vi "Edycja Wykres 1.vi"(8 "error in (no error)":errorcluster, 10 "Data in":T3) -> (0 "error out":errorcluster)   [LabVIEW 2014]
doc: "Program do edycji wykresów\ndodaje kursory, liczy odległość między kursorami pomiarowymi"
uses:
  Kontrolki/GUI/Wysw_kursorow_silver.ctl
  Kontrolki/Przetwarzanie/Kanaly.ctl
  Kontrolki/GUI/fx_przycisk.ctl
  Kontrolki/GUI/Edycja_blokowanie_free.ctl
  Kontrolki/Debug/Debug SigParam.ctl
  Kontrolki/Debug/DebugTyp.ctl
  <vilib>/Utility/miscctls.llb/LVCursorListTypeDef.ctl
  <vilib>/Utility/miscctls.llb/LVPointTypeDef.ctl
  Kontrolki/GUI/Edycja Leg Ctrl.ctl
  Kontrolki/FVGs/FVG akcje podstawowa.ctl
  <vilib>/measure/NI_MABase.lvlib
panel:
  out "Cluster":T1
  in  "Zablokowane free out":T2[](array[typedef])
  in  "Array":T4(array[cluster])=[{"signal type"=enum."Sine Wave", "frequency"=10.0, "amplitude"=2.0}, {"signal type"=enum."Sine Wave", "frequency"=13.0, "amplitude"=1.0}, {"signal type"=enum."Sine Wave", "frequency"=7.0, "amplitude"=1.0}, {"signal type"=enum."Sine Wave", "frequency"=5.0, "amplitude"=3.0}] {"amplitude" format="%0.2p"; "frequency" format="%0.2p"}
  in  "Kursory":i32(listbox)
  in  "Tab Control":T5(tab)
  out "Wykres 1":waveform(dbl)[](graph)
  out "Wykres 3":waveform(dbl)[](graph)
  out "Wykres 2":waveform(dbl)[](graph)
  out "XY Graph":cluster{"Y":dbl[], "Y":dbl[]}(graph)
  in  "Przebieg Y":string(combo)
  in  "Przebieg X":string(combo)
  out "Parametry out":T6
  out "Data in 2":T3
  out "Przebiegi Wfm":waveform(dbl)[](array[waveform])
  in  "KursOkno":bool
  in  "Edytuj_kur":bool
  in  "Funkcja":T8
  in  "Zapisz rys":bool
  in  "Save Wykres":bool
  in  "Pomiarowe Kursor":bool
  in  "Remove Kursor":bool
  in  "Add Kursor":bool
  in  "Stop":bool
  # "UWAGA!"
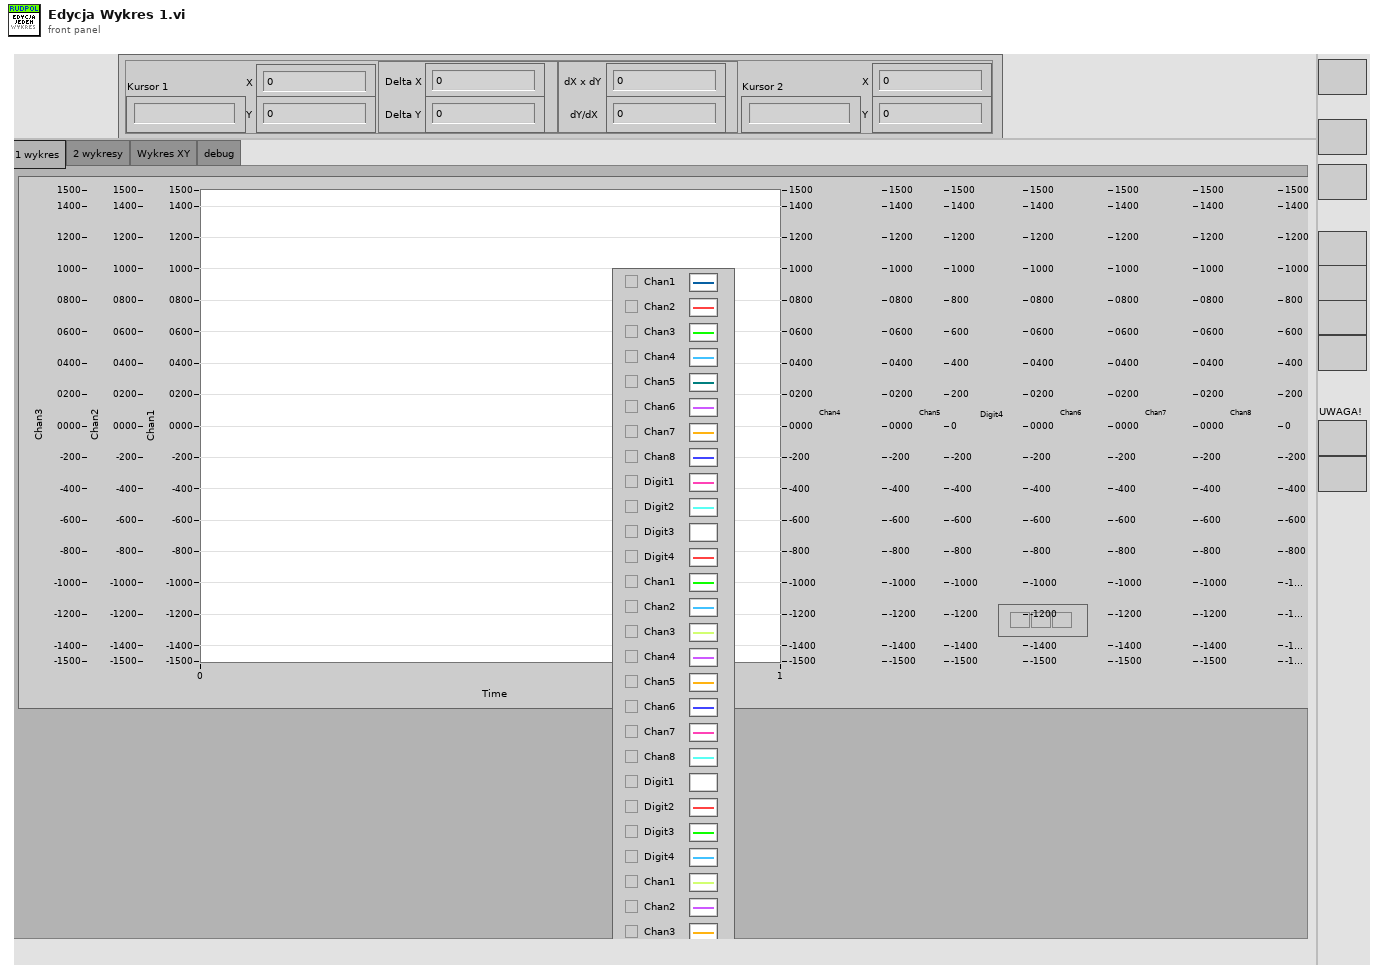
[diagram p1: front panel]
types:
  T1 = typedef "Wysw_kursorow_silver.ctl" = cluster{"Nazwa.1":string, "Nazwa.2":string, "Pos.X1":dbl, "Pos.Y1":dbl, "Delta.X":dbl, "Delta.Y":dbl, "Pos.X2":dbl, "Pos.Y2":dbl, "iloczyn dXY":dbl, "IlorazdYX":dbl}
  T2 = typedef "Edycja_blokowanie_free.ctl" = cluster{"Pozycja Y":dbl, "Pozycja X":dbl, "BlokujX":bool, "BlokujY":bool, "Zablokowane":i32}
  T3 = typedef "Kanaly.ctl" = cluster{"Analogowe":waveform(dbl)[], "Cyfrowe":waveform(dbl)[], "Zwarcie":waveform(dbl)[], "Enkoder":waveform(dbl)[]}
  T4 = cluster{"signal type":enum16{"Sine Wave", "Triangle Wave", "Square Wave", "Sawtooth Wave"}, "frequency":dbl, "amplitude":dbl}[]
  T5 = enum32{"1 wykres", "2 wykresy", "Wykres XY", "debug"}
  T6 = typedef "Debug SigParam.ctl" = cluster{"Analog":T7, "Digital":T7, "Enkoder":T7}
  T7 = typedef "DebugTyp.ctl" = cluster{"Liczba Kan":i32, "Nazwy":string[], "Rozm":i32, "dt":dbl}
  T8 = typedef "fx_przycisk.ctl" = bool
  T9 = enum16{"Sine Wave", "Triangle Wave", "Square Wave", "Sawtooth Wave"}
  T10 = typedef "Edycja Leg Ctrl.ctl" = cluster{"Leg 1":bool, "Leg 2":bool, "Leg 3":bool}
  T11 = typedef "LVPointTypeDef.ctl" = cluster{"Horizontal":i16, "Vertical":i16}
  T12 = typedef "FVG akcje podstawowa.ctl" = enum16{"GET", "SET"}
  T13 = typedef "LVCursorListTypeDef.ctl" = cluster{"Name":string, "Color":u32, "Style":u8, "Point Style":u8, "Name Visible":bool, "Allow Drag":bool, "Cursor Mode":u32, "Plot":i32, "Index":i32, "Position":cluster{"X":dbl, "Y":dbl}, "X Scale":u32, "Y Scale":u32, "Watch Plots":i32[], "Watch All Plots":bool, "Plot Area":i32, "Label Offset":cluster{"X":dbl, "Y":dbl}}[]
  T14 = typedef "LVBoundsTypeDef.ctl" = cluster{"Width":u32, "Height":u32}
  T15 = typedef "dwa_przebiegi_.ctl" = cluster{"Plot1":i32, "Plot2":i32}
  T16 = typedef "LVPoint32TypeDef.ctl" = cluster{"Horizontal":i32, "Vertical":i32}
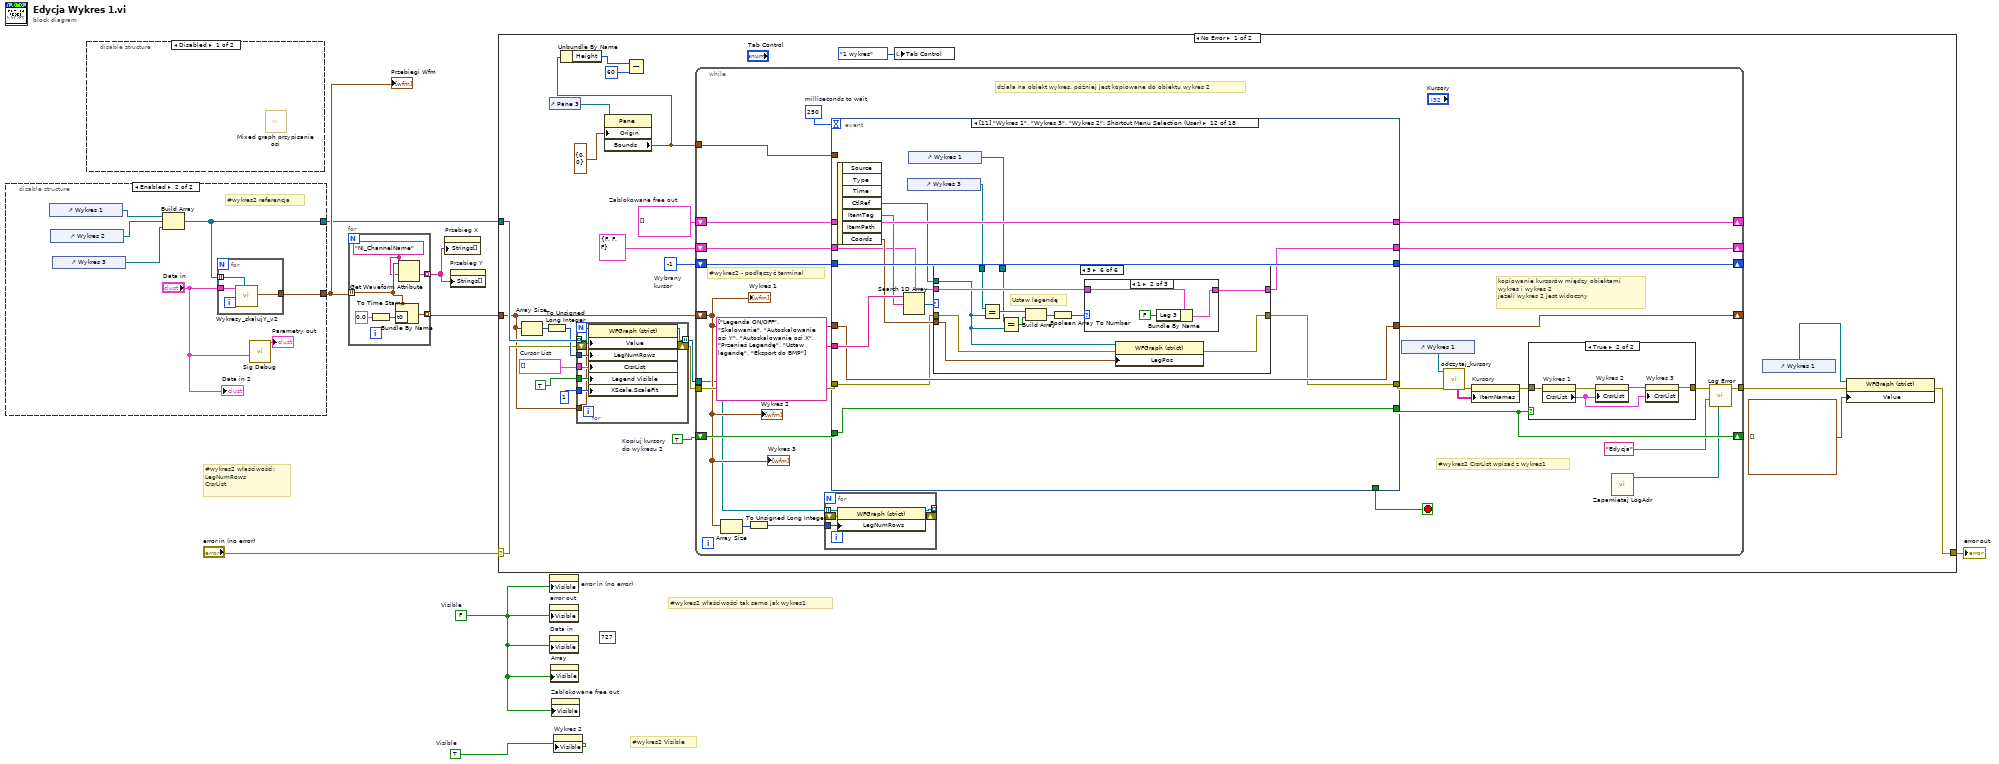
[diagram p0: block diagram]
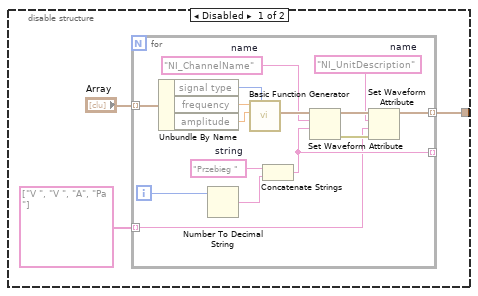
[diagram p3: hidden frame]
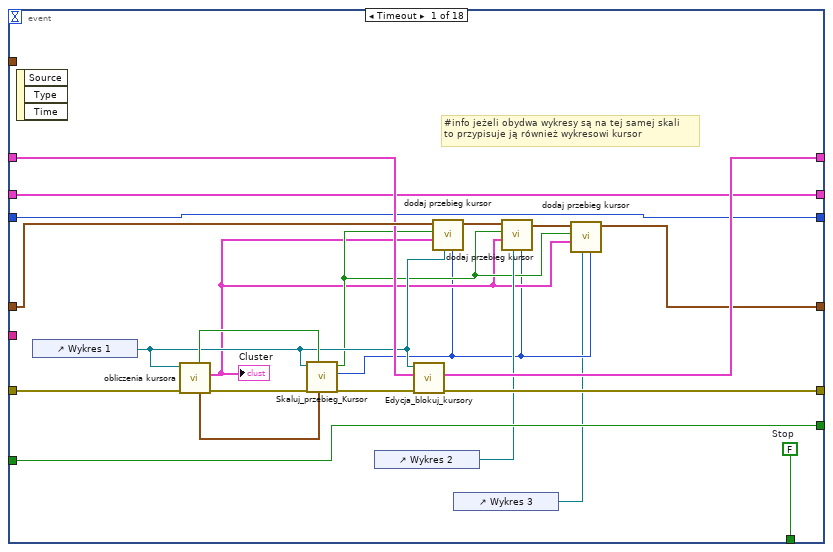
[diagram p5: hidden frame]
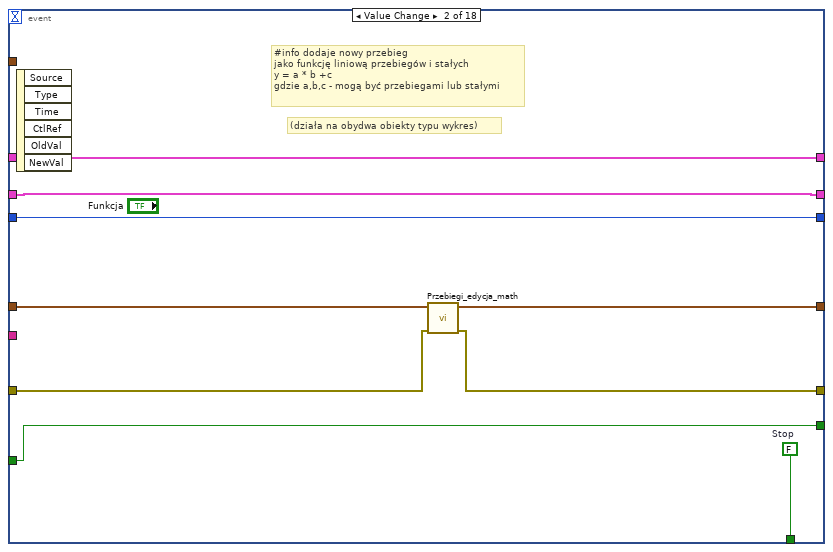
[diagram p6: hidden frame]
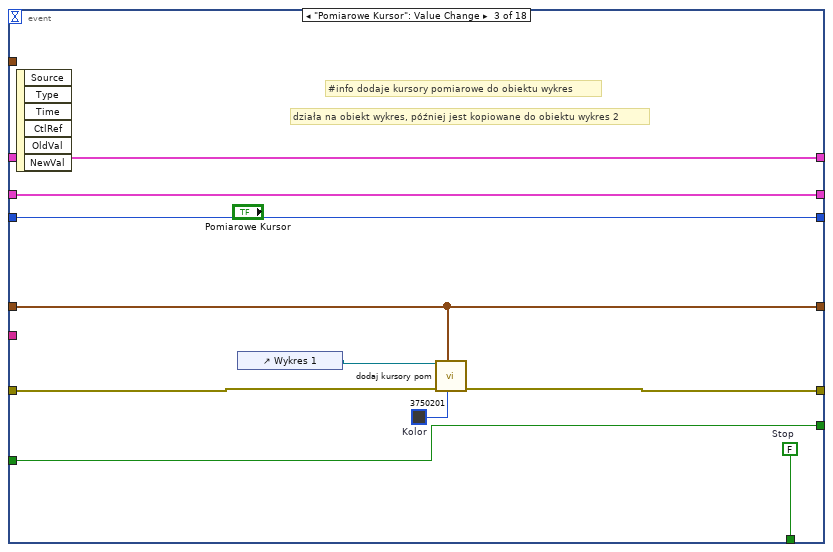
[diagram p7: hidden frame]
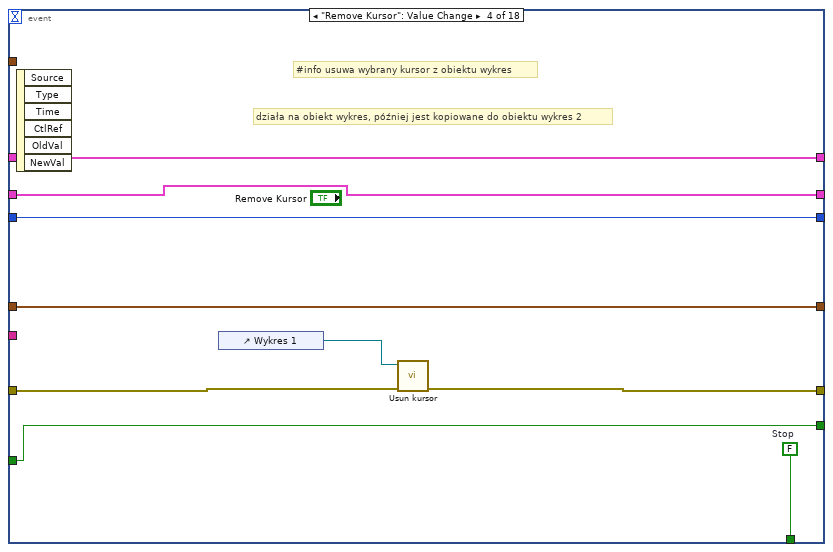
[diagram p8: hidden frame]
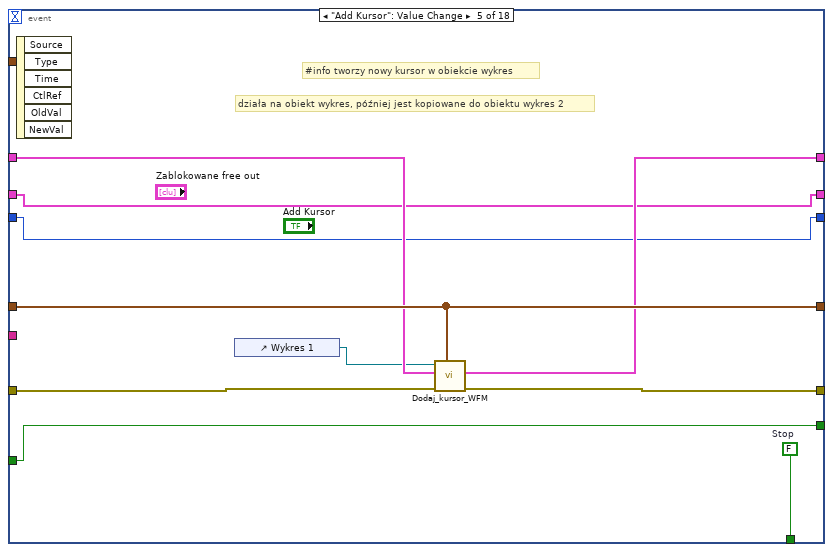
[diagram p9: hidden frame]
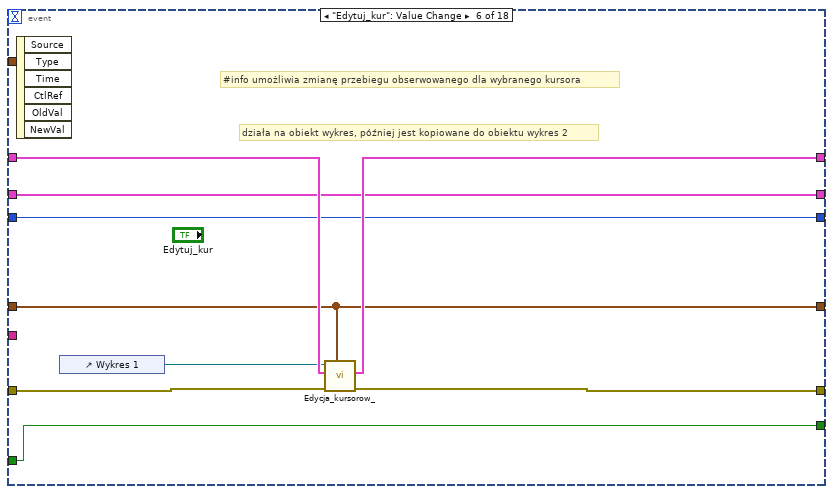
[diagram p10: hidden frame]
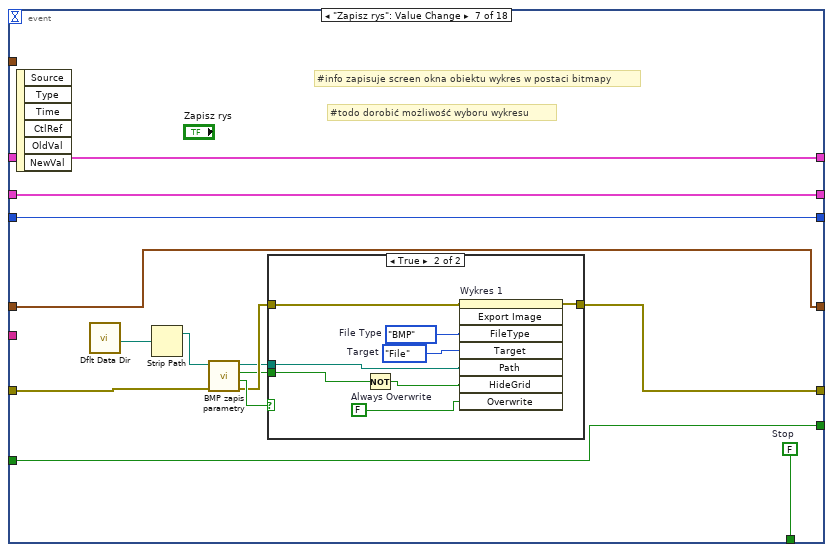
[diagram p11: hidden frame]
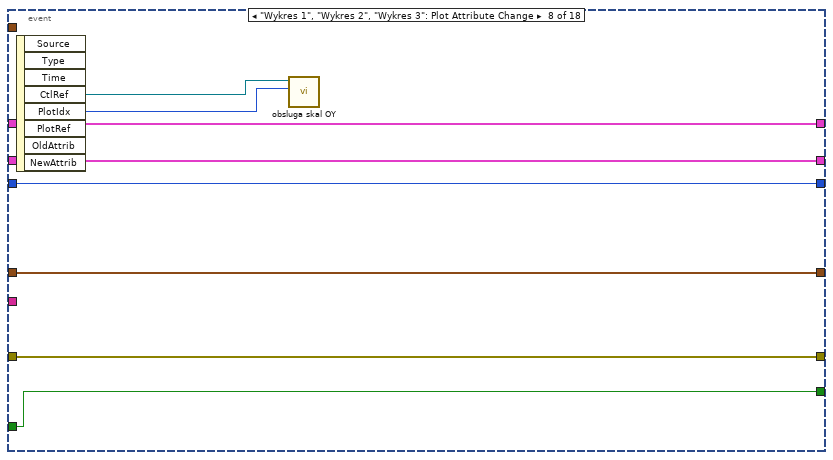
[diagram p13: hidden frame]
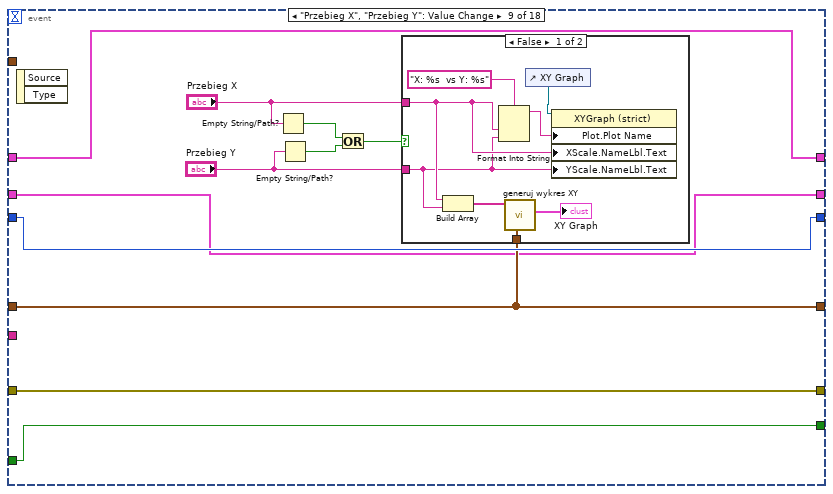
[diagram p14: hidden frame]
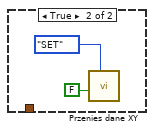
[diagram p15: hidden frame]
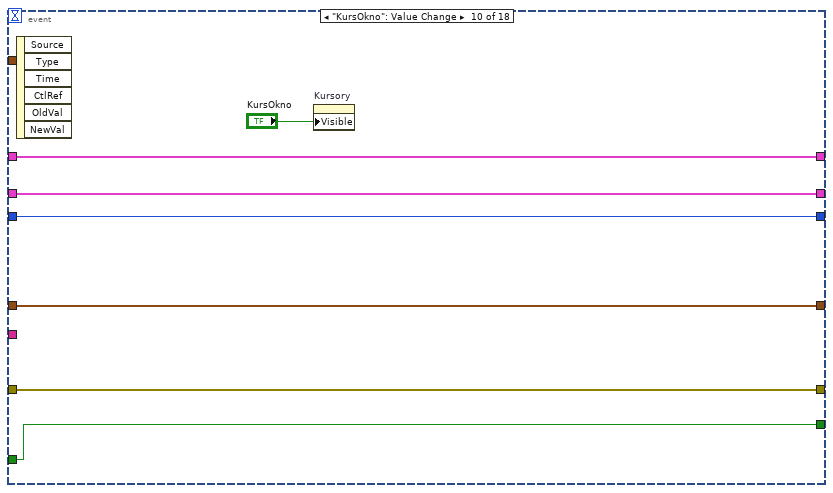
[diagram p16: hidden frame]
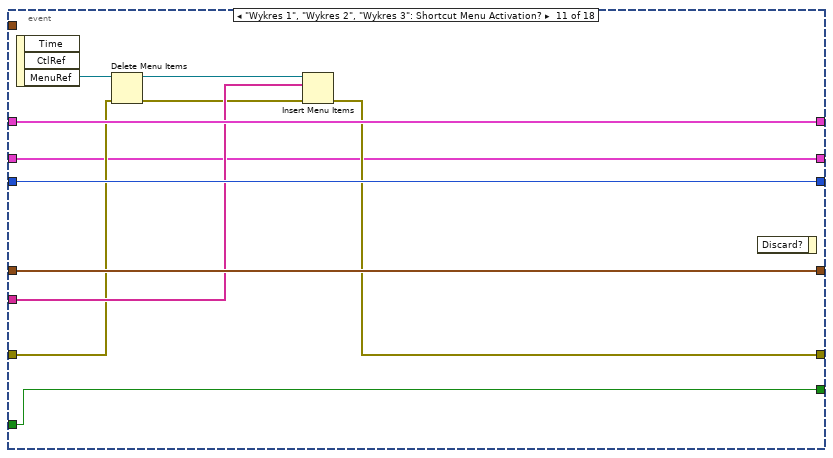
[diagram p17: hidden frame]
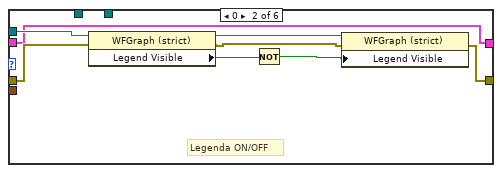
[diagram p19: hidden frame]
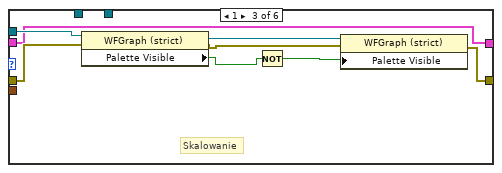
[diagram p20: hidden frame]
diagram:
  w3 = TRUE  # Visible
  (unwired) u32 727 ("Plot Area:Size:Width")
  w4 = FALSE  # Visible
  # "#wykres2 właściwości:\nLegNumRows\nCrsrList"
  # "#wykres2 Visible"
  # "#wykres2 właściwości tak samo jak wykres1"
  n1 = disable-structure shown="Enabled" {
    disable-tunnel: [w10 w28] -> w6
    disable-tunnel: [_ w27] -> w1
    frame Disabled {
      n2 = for {
        tunnel: "Array" -> [w23] mode=indexing
        tunnel: [w14] -> w10 mode=indexing
        tunnel: [w17] -> _ mode=indexing
        tunnel: string[] ["V ", "V ", "A", "Pa "] -> [w12] mode=indexing
        i -> [w18]
        w13 = "NI_UnitDescription"  # name
        w20 = "Przebieg "  # string
        w21 = "NI_ChannelName"  # name
        n3 = Unbundle By Name(w23) -> ("signal type"=w26:T9, "frequency"=w25:dbl, "amplitude"=w24:dbl)
        n4 = Number To Decimal String(number=w18) -> (decimal integer string=w19:string)  [unwired: 1 in]
        n5 = call <vilib>:"Basic Function Generator.vi"("signal type"=w26, "amplitude"=w24, "frequency"=w25) -> ("signal out"=w22:waveform(dbl))  [unwired: 6 in, 2 out]
        n6 = Concatenate Strings(w20, w19) -> (w17:string)
        n7 = Set Waveform Attribute(5:w17, 6:w21, 7:w22) -> (0:w16:errorcluster, 3:w15:waveform(dbl))  [unwired: 1 in, 1 out]
        n8 = Set Waveform Attribute(4:w16, 5:w12, 6:w13, 7:w15) -> (3:w14:waveform(dbl))  [unwired: 2 out]
      }
    }
    frame Enabled {
      # "#wykres2 referencja"
      n9 = control-ref of="Wykres 1"() -> (w31:refnum<vi>)
      n10 = control-ref of="Wykres 2"() -> (w30:refnum<vi>)
      n11 = control-ref of="Wykres 3"() -> (w29:refnum<vi>)
      n12 = Build Array(w31, w30, w29) -> (w27:refnum<vi>[])
      n13 = for {
        tunnel: "Data in" -> [w36]
        tunnel: [w35] -> w28
        tunnel: w27 -> [w34] mode=indexing
        n14 = call "Wykresy_skalujY_v2.vi"("Wvm Ref in"=w34, "Data in"=w36) -> ("Przebiegi Wfm"=w35:waveform(dbl)[])  [unwired: 7 in, 2 out]
      }
      n15 = call "Sig Debug.vi"("Kanaly in"="Data in") -> ("Parametry out"=→"Parametry out":T6)  [unwired: 8 in, 2 out]
      "Data in 2" <- "Data in"
    }
  }
  "Przebiegi Wfm" <- w6
  n16 = disable-structure shown="Disabled" {
    frame Disabled {
      n17 = call "Mixed graph przypisanie osi.vi"() -> ()  [unwired: 9 in, 3 out]
    }
    frame Enabled {
    }
  }
  n18 = for {
    tunnel: w6 -> [w39] mode=indexing
    tunnel: [w42] -> w5 mode=indexing
    tunnel: [w37] -> w2 mode=indexing
    w38 = "NI_ChannelName" ("name")
    n19 = To Time Stamp(1:0.0) -> (0:w40:timestamp)
    n20 = Bundle By Name(cluster=w39, "t0"=w40) -> (w42:waveform(dbl))
    n21 = Get Waveform Attribute(5:w38, 6:w38, 7:w39) -> (1:w37:string)  [unwired: 1 in, 3 out]
  }
  n22 = property on="Przebieg X" class="CmbBox"("Strings[]"=w2) -> ()  [unwired: 2 in, 2 out]
  n23 = property on="Przebieg Y" class="CmbBox"("Strings[]"=w2) -> ()  [unwired: 2 in, 2 out]
  n24 = case shown="No Error" "error in (no error)" {
    selector: "error in (no error)" -> [w50 w420]
    tunnel: [w61 w420] -> w7
    tunnel: w5 -> [w44 _]
    tunnel: w1 -> [w52 _]
    frame No Error {
      w63 = TRUE  # Kopiuj kursory do wykresu 2
      w64 = -1  # Wybrany kursor
      w65 = T2[] []  # Zablokowane free out
      w48 = T13 []  # Cursor List
      n25 = Array Size(array=w44) -> (size(s)=w66:i32)
      n26 = To Unsigned Long Integer(number=w66) -> (unsigned 32bit integer=w51:u32)
      n27 = control-ref of="Pane 3"() -> (w59:refnum<vi>)
      n28 = for {
        tunnel: w52 -> [w74] mode=indexing
        tunnel: w51 -> [w73]
        shift-right: [w72] -> w49
        shift-left: w50 -> [_]
        tunnel: w48 -> [w71]
        tunnel: [w70] -> w47 mode=indexing
        tunnel: u8 1 ("X Scale.Scale Fit") -> [w69]
        tunnel: TRUE ("Legend:Visible") -> [w68]
        tunnel: w44 -> [w67]
        n29 = property class="WFGraph (strict)"(reference=w74, "Value"=w67, "LegNumRows"=w73, "CrsrList"=w71, "Legend Visible"=w68, "XScale.ScaleFit"=w69) -> (reference out=w70:refnum<vi>, error out=w72:errorcluster)  [unwired: 1 in]
      }
      n30 = property class="Pane"(reference=w59, "Origin"=T11 {"Horizontal"=0, "Vertical"=0}) -> ("Bounds"=w56:T14)  [unwired: 1 in, 2 out]
      n31 = Unbundle By Name(w56) -> ("Height"=w55:u32)
      n32 = Subtract(x=w55, y=u32 60) -> ()  [unwired: 1 out]
      n33 = while {
        tunnel: w49 -> [w101]
        tunnel: [w85] -> w62
        shift-right: [w98] -> _
        shift-left: w44 -> [w79]
        shift-right: [w97] -> _
        shift-left: w65 -> [w96]
        shift-right: [w91] -> _
        shift-left: w64 -> [w92]
        shift-right: [w88] -> _
        shift-left: w63 -> [w89]
        tunnel: w56 -> [w83]
        tunnel: w47 -> [w77]
        shift-right: [w75] -> _
        shift-left: T10 {"Leg 1"=FALSE, "Leg 2"=FALSE, "Leg 3"=FALSE} ("Legenda") -> [w76]
        stop <- w99 stop-if-true
        w100 = 250  # milliseconds to wait
        # "#wykres2 CrsrList wpisać z wykres1"
        # "#wykres2 - podłączyć terminal"
        # "kopiowanie kursorów między obiektami\nwykres i wykres 2\njeżeli wykres 2 jest widoczny"
        # "działa na obiekt wykres, później jest kopiowane do obiektu wykres 2"
        n34 = Array Size(array=w79) -> (size(s)=w87:i32)
        n35 = To Unsigned Long Integer(number=w87) -> (unsigned 32bit integer=w78:u32)
        n36 = for {
          tunnel: w77 -> [w106] mode=indexing
          tunnel: w78 -> [w105]
          shift-right: [w103] -> _
          shift-left: _ -> [w104]
          tunnel: [w102] -> _ mode=indexing
          n37 = property class="WFGraph (strict)"(reference=w106, error in=w104, "LegNumRows"=w105) -> (reference out=w102:refnum<vi>, error out=w103:errorcluster)
        }
        n38 = event shown="[11] \"Wykres 1\", \"Wykres 3\", \"Wykres 2\": Shortcut Menu Selection (User)" {
          selector: _ -> [_ _ _ _ _ _ _ _ _ _ _ _ _ _ _ _ _ _]
          dyn-events: _ -> [_ _ _ _ _ _ _ _ _ _ _ _ _ _ _ _ _ _]
          timeout: w100 -> [_ _ _ _ _ _ _ _ _ _ _ _ _ _ _ _ _ _]
          tunnel: w79 -> [w131 w142 w150 w158 w170 w176 w185 w210 w213 w238 w250 w258 w340 w359 w368 w378 w411 w417]
          tunnel: w101 -> [w133 w140 w152 w161 w171 w178 w191 w211 w222 w239 w242 w256 w345 w360 w363 _ w412 w418]
          tunnel: [w126 w139 w151 w160 w166 w177 w194 w211 w222 w239 w241 w255 w344 w360 w362 w375 w412 w418] -> w94
          tunnel: [w132 w138 w148 w159 w169 _ w193 _ _ _ _ _ _ _ w367 _ _ "Stop"] -> w99
          tunnel: [w119 w141 w150 w158 w170 w176 w185 w210 w213 w238 w250 w258 w340 w359 w368 w378 w411 w417] -> w98
          tunnel: [w128 w137 w147 w157 w167 w179 w184 w209 w221 w237 w249 w265 w349 w358 w366 w377 w410 w416] -> w97
          tunnel: w96 -> [w129 w137 w147 w157 w168 w180 w184 w209 w221 w237 w249 w265 w349 w358 w366 w377 w410 w416]
          tunnel: w92 -> [w124 w136 w146 w156 w165 w175 w183 w208 w220 w236 w248 w264 w348 _ w365 w374 _ w415]
          tunnel: [w124 w136 w146 w156 w165 w175 w183 w208 w220 w236 w248 w264 w348 w357 w365 w374 w409 w415] -> w91
          tunnel: [w123 w135 w145 w155 w164 w174 w182 w207 w219 w235 w247 w263 w347 w356 w364 w370 w408 w414] -> w88
          tunnel: w89 -> [w123 w135 w145 w155 w164 w174 w182 w207 w219 w235 w247 w263 w347 w356 w364 w370 w408 w414]
          tunnel: w83 -> [_ _ _ _ _ _ _ _ _ _ _ _ _ _ _ _ _ _]
          tunnel: string[] ["Legenda ON/OFF", "Skalowanie", "Autoskalowanie osi Y", "Autoskalowanie osi X", "Przenieś Legendę", "Ustaw legendę", "Eksport do BMP"] -> [_ _ _ _ _ _ _ _ _ _ w246 w262 _ _ _ _ _ _]
          tunnel: w76 -> [w113 w134 w143 w153 w162 w172 w181 w204 w212 w233 w240 w252 w339 w355 w361 w369 w407 w413]
          tunnel: [w113 w134 w143 w153 w162 w172 w181 w204 w212 w233 w240 w251 w339 w355 w361 w369 w407 w413] -> w75
          event Timeout {
            w132 = FALSE  # Stop
            # "#info jeżeli obydwa wykresy są na tej samej skali\nto przypisuje ją również wykresowi kursor"
            n39 = event-data() -> ()  [unwired: 1 in, 3 out]
            n40 = control-ref of="Wykres 1"() -> (w122:refnum<vi>)
            n41 = call "obliczenia kursora.vi"("error in (no error)"=w133, "Wykres Ref"=w122) -> ("error out"=w130:errorcluster, "Data"=w116:T1, "Przebiegi Monit"=w127:T15, "Pomiarowe OK?"=w125:bool)  [unwired: 6 in]
            "Cluster" <- w116
            n42 = call "Skaluj_przebieg_Kursor.vi"("Przebiegi Monit"=w127, "Pomiarowe OK? in"=w125, "WaveformGraph in"=w122) -> ("Plot.YScaleIdx"=w115:u32, "Pomiarowe OK? out"=w117:bool)  [unwired: 6 in, 1 out]
            n43 = control-ref of="Wykres 2"() -> (w120:refnum<vi>)
            n44 = call "Edycja_blokuj_kursory.vi"("error in (no error)"=w130, "Zablokowane free in"=w129, "Wykres Ref"=w122) -> ("error out"=w126:errorcluster, "Zablokowane free out"=w128:T2[])  [unwired: 7 in]
            n45 = call "dodaj przebieg kursor.vi"("Plot.Y Scale Index"=w115, "WaveformGraph in"=w122, "Data"=w116, "Pomiarowe OK?"=w117, "Przebiegi in"=w131) -> ("przebiegi out"=w121:waveform(dbl)[])  [unwired: 5 in, 1 out]
            n46 = control-ref of="Wykres 3"() -> (w114:refnum<vi>)
            n47 = call "dodaj przebieg kursor.vi"("Plot.Y Scale Index"=w115, "WaveformGraph in"=w120, "Data"=w116, "Pomiarowe OK?"=w117, "Przebiegi in"=w121) -> ("przebiegi out"=w118:waveform(dbl)[])  [unwired: 5 in, 1 out]
            n48 = call "dodaj przebieg kursor.vi"("Plot.Y Scale Index"=w115, "WaveformGraph in"=w114, "Data"=w116, "Pomiarowe OK?"=w117, "Przebiegi in"=w118) -> ("przebiegi out"=w119:waveform(dbl)[])  [unwired: 5 in, 1 out]
          }
          event Value Change {
            w138 = FALSE  # Stop
            # "(działa na obydwa obiekty typu wykres)"
            # "#info dodaje nowy przebieg\njako funkcję liniową przebiegów i stałych\ny = a * b +c\ngdzie a,b,c - mogą być przebiegami lub stałymi"
            n49 = event-data() -> ()  [unwired: 1 in, 6 out]
            n50 = call "Przebiegi_edycja_math.vi"("error in (no error)"=w140, "Wektor przebiegow in"=w142) -> ("error out"=w139:errorcluster, "Wektor przebiegow out"=w141:waveform(dbl)[])  [unwired: 8 in]
          }
          event "Pomiarowe Kursor": Value Change {
            w148 = FALSE  # Stop
            w149 = u32 3750201  # Kolor
            # "działa na obiekt wykres, później jest kopiowane do obiektu wykres 2"
            # "#info dodaje kursory pomiarowe do obiektu wykres"
            n51 = event-data() -> ()  [unwired: 1 in, 6 out]
            n52 = control-ref of="Wykres 1"() -> (w144:refnum<vi>)
            n53 = call "dodaj kursory pom.vi"("Kolor"=w149, "Wektor przebiegow"=w150, "error in (no error)"=w152, "Wykres Ref"=w144) -> ("error out"=w151:errorcluster)  [unwired: 7 in]
          }
          event "Remove Kursor": Value Change {
            w159 = FALSE  # Stop
            # "#info usuwa wybrany kursor z obiektu wykres"
            # "działa na obiekt wykres, później jest kopiowane do obiektu wykres 2"
            n54 = event-data() -> ()  [unwired: 1 in, 6 out]
            n55 = control-ref of="Wykres 1"() -> (w154:refnum<vi>)
            n56 = call "Usun kursor.vi"("error in (no error)"=w161, "Wykres Ref"=w154) -> ("error out"=w160:errorcluster)  [unwired: 9 in]
          }
          event "Add Kursor": Value Change {
            w169 = FALSE  # Stop
            # "działa na obiekt wykres, później jest kopiowane do obiektu wykres 2"
            # "#info tworzy nowy kursor w obiekcie wykres"
            n57 = event-data() -> ()  [unwired: 1 in, 6 out]
            n58 = control-ref of="Wykres 1"() -> (w163:refnum<vi>)
            n59 = call "Dodaj_kursor_WFM.vi"("Wektor przebiegow"=w170, "error in (no error)"=w171, "Zablokowane free in"=w168, "Wykres Ref"=w163) -> ("error out"=w166:errorcluster, "Zablokowane free out"=w167:T2[])  [unwired: 6 in]
          }
          event "Edytuj_kur": Value Change {
            # "#info umożliwia zmianę przebiegu obserwowanego dla wybranego kursora"
            # "działa na obiekt wykres, później jest kopiowane do obiektu wykres 2"
            n60 = event-data() -> ()  [unwired: 1 in, 6 out]
            n61 = control-ref of="Wykres 1"() -> (w173:refnum<vi>)
            n62 = call "Edycja_kursorow_.vi"("Wykres"=w176, "error in (no error)"=w178, "Zablokowane free in"=w180, "Wykres Ref"=w173) -> ("error out"=w177:errorcluster, "Zablokowane free out"=w179:T2[])  [unwired: 6 in]
          }
          event "Zapisz rys": Value Change {
            w193 = FALSE  # Stop
            # "#todo dorobić możliwość wyboru wykresu"
            # "#info zapisuje screen okna obiektu wykres w postaci bitmapy"
            n63 = event-data() -> ()  [unwired: 1 in, 6 out]
            n64 = call <vilib>:"Dflt Data Dir.vi"() -> ("App:Default Data Directory"=w186:path)
            n65 = Strip Path(path=w186) -> (stripped path=w187:path)  [unwired: 1 out]
            n66 = call "BMP zapis parametry.vi"("error in (no error)"=w191, "Katalog"=w187) -> ("error out"=w190:errorcluster, "OK?"=w192:bool, "linie out"=w188:bool, "Katalog out"=w189:path)  [unwired: 6 in]
            n67 = case shown="True" w192 {
              tunnel: w190 -> [w195 w202]
              tunnel: [w195 w196] -> w194
              tunnel: w189 -> [_ w199]
              tunnel: w188 -> [_ w203]
              frame False {
              }
              frame True {
                w197 = FALSE  # Always Overwrite
                w200 = enum32{"File", "Clipboard"}."File"  # Target
                w201 = enum32{"BMP", "EPS", "EMF", "PICT"}."BMP"  # File Type
                n68 = Not(x=w203) -> (.not. x?=w198:bool)
                n69 = invoke on="Wykres 1" class="WFGraph (strict)" method="Export Image"(error in=w202, "FileType"=w201, "Target"=w200, "Path"=w199, "HideGrid"=w198, "Overwrite"=w197) -> (error out=w196:errorcluster)  [unwired: 2 in, 7 out]
              }
            }
          }
          event "Wykres 1", "Wykres 2", "Wykres 3": Plot Attribute Change {
            n70 = event-data() -> ("CtlRef"=w206:refnum<vi>, "PlotIdx"=w205:i32)  [unwired: 1 in, 6 out]
            n71 = call "obsluga skal OY.vi"("PlotIdx"=w205, "WaveformGraph in"=w206) -> ()  [unwired: 9 in, 1 out]
          }
          event "Przebieg X", "Przebieg Y": Value Change {
            n72 = event-data() -> ()  [unwired: 1 in, 2 out]
            n73 = Empty String/Path?(string/path="Przebieg X") -> (empty?=w216:bool)
            n74 = Empty String/Path?(string/path="Przebieg Y") -> (empty?=w217:bool)
            n75 = Or(x=w216, y=w217) -> (x .or. y?=w218:bool)
            n76 = case shown="False" w218 {
              tunnel: "Przebieg X" -> [w228 _]
              tunnel: "Przebieg Y" -> [w227 _]
              tunnel: w213 -> [w223 _]
              frame False {
                n77 = Build Array(w228, w227) -> (w226:string[])
                n78 = Format Into String(format string="X: %s  vs Y: %s", w228, w227) -> (resulting string=w229:string)  [unwired: 2 in, 1 out]
                n79 = call "generuj wykres XY.vi"("Przebiegi Wfm"=w223, "Wykresy out"=w226) -> ("output cluster"=→"XY Graph":cluster{"Y":dbl[], "Y":dbl[]})  [unwired: 8 in, 1 out]
                n80 = control-ref of="XY Graph"() -> (w224:refnum<vi>)
                n81 = property on="Property Node" class="XYGraph (strict)"(reference=w224, "Plot.Plot Name"=w229, "XScale.NameLbl.Text"=w228, "YScale.NameLbl.Text"=w227) -> ()  [unwired: 1 in, 2 out]
              }
              frame True {
                n82 = call "Przenies dane XY.vi"("Akcja (GET)"=FVG_akcje_podstawowa."SET", "Rysuj in"=FALSE) -> ()  [unwired: 7 in, 3 out]
              }
            }
          }
          event "KursOkno": Value Change {
            n83 = event-data() -> ()  [unwired: 1 in, 6 out]
            n84 = property on="Kursory" class="MCListbox (strict)"("Visible"="KursOkno") -> ()  [unwired: 2 in, 2 out]
          }
          event "Wykres 1", "Wykres 2", "Wykres 3": Shortcut Menu Activation? {
            n85 = event-data() -> ("MenuRef"=w245:refnum<k9>)  [unwired: 1 in, 2 out]
            n86 = Delete Menu Items(6:w242, 9:w245) -> (0:w243:errorcluster, 3:w244:refnum<k9>)  [unwired: 2 in]
            n87 = Insert Menu Items(6:w243, 8:w246, 9:w244) -> (0:w241:errorcluster)  [unwired: 3 in, 2 out]
            n88 = event-data() -> ()  [unwired: 2 in, 1 out]
          }
          event "Wykres 1", "Wykres 3", "Wykres 2": Shortcut Menu Selection (User) {
            n89 = event-data() -> ("CtlRef"=w259:refnum<vi>, "ItemTag"=w261:string, "Coords"=w257:T16)  [unwired: 1 in, 4 out]
            n90 = Search 1D Array(1D array=w262, element=w261) -> (index of element=w260:i32)  [unwired: 1 in]
            n91 = control-ref of="Wykres 3"() -> (w253:refnum<vi>)
            n92 = control-ref of="Wykres 1"() -> (w254:refnum<vi>)
            n93 = case shown="5" w260 {
              tunnel: w259 -> [_ w275 w283 w288 w297 w311]
              tunnel: w257 -> [_ _ _ _ _ w309]
              tunnel: w256 -> [w267 w270 w278 w286 w295 w310]
              tunnel: [w267 w269 w277 w285 w295 w308] -> w255
              tunnel: w252 -> [w266 w268 w276 w284 w290 w315]
              tunnel: w254 -> [_ _ _ _ w296 w312]
              tunnel: w253 -> [_ _ _ _ w298 w313]
              tunnel: [w266 w268 w276 w284 w289 w314] -> w251
              frame -1, Default {
                # "nie rób nic - nieaktywna opcja pop up menu"
              }
              frame 0 {
                # "Legenda ON/OFF"
                n94 = property class="WFGraph (strict)"(reference=w275, error in=w270) -> (reference out=w272:refnum<vi>, error out=w273:errorcluster, "Legend Visible"=w271:bool)
                n95 = Not(x=w271) -> (.not. x?=w274:bool)
                n96 = property class="WFGraph (strict)"(reference=w272, error in=w273, "Legend Visible"=w274) -> (error out=w269:errorcluster)  [unwired: 1 out]
              }
              frame 1 {
                # "Skalowanie"
                n97 = property class="WFGraph (strict)"(reference=w283, error in=w278) -> (reference out=w280:refnum<vi>, error out=w279:errorcluster, "Palette Visible"=w282:bool)
                n98 = Not(x=w282) -> (.not. x?=w281:bool)
                n99 = property class="WFGraph (strict)"(reference=w280, error in=w279, "Palette Visible"=w281) -> (error out=w277:errorcluster)  [unwired: 1 out]
              }
              frame 3 {
                # "Autoskalowanie osi X"
                n100 = property class="WFGraph (strict)"(reference=w288, error in=w286, "XScale.ScaleFit"=u8 1 ("X Scale.Scale Fit")) -> (error out=w285:errorcluster)  [unwired: 1 out]
              }
              frame 4 {
                # "Przenieś Legendę"
                n101 = Equal?(x=w298, y=w297) -> (x = y?=w294:bool)
                n102 = Equal?(x=w296, y=w297) -> (x = y?=w293:bool)
                n103 = Build Array(w294, w293) -> (w292:bool[])
                n104 = Boolean Array To Number(Boolean array=w292) -> (number=w291:u32)
                n105 = case shown="2" w291 {
                  tunnel: w290 -> [w301 w303 w306]
                  tunnel: [w300 w302 w305] -> w289
                  frame 0, Default {
                    n106 = Bundle By Name(cluster=w301, "Leg 2"=TRUE) -> (w300:T10)
                  }
                  frame 1 {
                    n107 = Bundle By Name(cluster=w303, "Leg 3"=TRUE ("Leg 2")) -> (w302:T10)
                  }
                  frame 2 {
                    n108 = Bundle By Name(cluster=w306, "Leg 1"=TRUE ("Leg 2")) -> (w305:T10)
                  }
                }
              }
              frame 5 {
                # "Ustaw legendę"
                n109 = Equal?(x=w313, y=w311) -> (x = y?=w319:bool)
                n110 = Equal?(x=w312, y=w311) -> (x = y?=w318:bool)
                n111 = Build Array(w319, w318) -> (w317:bool[])
                n112 = Boolean Array To Number(Boolean array=w317) -> (number=w316:u32)
                n113 = case shown="1" w316 {
                  tunnel: w315 -> [w322 w324 w327]
                  tunnel: [w321 w323 w326] -> w314
                  frame 0, Default {
                    n114 = Bundle By Name(cluster=w322, "Leg 2"=FALSE) -> (w321:T10)
                  }
                  frame 1 {
                    n115 = Bundle By Name(cluster=w324, "Leg 3"=FALSE ("Leg 2")) -> (w323:T10)
                  }
                  frame 2 {
                    n116 = Bundle By Name(cluster=w327, "Leg 1"=FALSE ("Leg 2")) -> (w326:T10)
                  }
                }
                n117 = property class="WFGraph (strict)"(reference=w311, error in=w310, "LegPos"=w309) -> (error out=w308:errorcluster)  [unwired: 1 out]
              }
            }
          }
          event "Wykres 1", "Wykres 2", "Wykres 3": Mouse Move {
            n118 = event-data() -> ("CtlRef"=w341:refnum<vi>, "Coords"=w346:T16)  [unwired: 1 in]
            n119 = control-ref of="Wykres 3"() -> (w343:refnum<vi>)
            n120 = control-ref of="Wykres 1"() -> (w342:refnum<vi>)
            n121 = Equal?(x=w341, y=w343) -> (x = y?=w335:bool)
            n122 = Equal?(x=w341, y=w342) -> (x = y?=w336:bool)
            n123 = Unbundle By Name(w339) -> ("Leg 1"=w338:bool, "Leg 3"=w337:bool, "Leg 2"=w333:bool)
            n124 = Not Or(1:w335, 2:w336) -> (0:w334:bool)
            n125 = And(x=w338, y=w336) -> (x .and. y?=w332:bool)
            n126 = And(x=w337, y=w335) -> (x .and. y?=w331:bool)
            n127 = And(x=w333, y=w334) -> (x .and. y?=w330:bool)
            n128 = Compound Arithmetic op=OR(w332, w331, w330) -> (w329:bool)
            n129 = case shown="True" w329 {
              tunnel: w341 -> [_ w354]
              tunnel: w345 -> [w350 w353]
              tunnel: w346 -> [_ w352]
              tunnel: [w350 w351] -> w344
              frame False {
              }
              frame True {
                n130 = property class="WFGraph (strict)"(reference=w354, error in=w353, "LegPos"=w352) -> (error out=w351:errorcluster)  [unwired: 1 out]
              }
            }
          }
          event "Kursory": Value Change {
            # "#info zapamiętuje ostatni wybrany kursor w obiekcie Kursory\ndo przesuwania scrollem"
            n131 = event-data() -> ("NewVal"=w357:i32)  [unwired: 1 in, 5 out]
          }
          event "Save Wykres": Value Change {
            w367 = FALSE  # Stop
            # "#info zapisuje dane z obiektu wykres do Excella"
            n132 = event-data() -> ()  [unwired: 1 in, 6 out]
            n133 = invoke on="Wykres 1" class="WFGraph (strict)" method="Export Data to Excel"(error in=w363) -> (error out=w362:errorcluster)  [unwired: 2 in, 2 out]
          }
          event "Wykres 1", "Wykres 2": Mouse Wheel {
            # "#todo obsługuje tylko kursory pojedyncze"
            # "#info obsługa scrolla dla kursorów w obiektach wykres i wykres 2"
            n134 = event-data() -> ("Delta"=w376:i32)  [unwired: 1 in, 1 out]
            n135 = property on="Wykres 1" class="WFGraph (strict)"("Active Cursor"=w374) -> (error out=w372:errorcluster, "Cursor.CursorMode"=w373:u32, "Cursor"=w371:refnum<vi>)  [unwired: 2 in, 1 out]
            n136 = case shown="1, Default" w373 {
              tunnel: w376 -> [w381 w391]
              tunnel: w372 -> [w385 w389]
              tunnel: w371 -> [w386 w388]
              tunnel: [w382 w387] -> w375
              frame 1, Default {
                n137 = property class="Curs"(reference=w386, error in=w385) -> (reference out=w383:refnum<vi>, error out=w384:errorcluster, "Cursor Index"=w380:i32)
                n138 = Subtract(x=w380, y=w381) -> (x-y=w379:i32)
                n139 = property class="Curs"(reference=w383, error in=w384, "Cursor Index"=w379) -> (error out=w382:errorcluster)  [unwired: 1 out]
              }
              frame 2 {
                n140 = property class="Curs"(reference=w388, error in=w389) -> (reference out=w393:refnum<vi>, error out=w392:errorcluster, "WatchPlots"=w390:i32[])
                n141 = for {
                  tunnel: w393 -> [w403]
                  tunnel: w392 -> [w402]
                  tunnel: w391 -> [w397]
                  tunnel: w390 -> [w396] mode=indexing
                  tunnel: [w394] -> w387
                  n142 = property class="Curs"(reference=w403, error in=w402, "Cursor Plot"=w396) -> (reference out=w401:refnum<vi>, error out=w400:errorcluster, "Cursor Index"=w399:i32)
                  n143 = Subtract(x=w399, y=w397) -> (x-y=w398:i32)
                  n144 = property class="Curs"(reference=w401, error in=w400, "Cursor Index"=w398) -> (error out=w395:errorcluster)  [unwired: 1 out]
                  n145 = case shown="No Error" w395 {
                    selector: w395 -> [w404 w406]
                    tunnel: [w404 w406] -> w394
                    frame No Error {
                      n146 = Wait (ms)(milliseconds to wait=u32 0) -> ()  [unwired: 1 out]
                    }
                    frame Error {
                    }
                  }
                }
              }
            }
          }
          event "Wykres 1", "Wykres 2": Cursor Release {
            # "#info wybiera ostatnio naciśnięty kursor\nw obiekcie wykres lub wykres 2 do obsługi scrolla"
            n147 = event-data() -> ("CursIdx"=w409:i32)  [unwired: 1 in, 3 out]
          }
          event "Stop": Value Change {
            # "#info obsługa przycisku STOP - zatrzymanie programu"
            n148 = event-data() -> ()  [unwired: 1 in, 6 out]
          }
        }
        n149 = control-ref of="Wykres 1"() -> (w80:refnum<vi>)
        n150 = call "odczytaj_kursory.vi"("error in (no error)"=w94, "WaveformGraph in"=w80) -> ("error out"=w95:errorcluster, "Array"=w93:string[][])  [unwired: 8 in]
        n151 = property on="Kursory" class="MCListbox (strict)"(error in=w95, "ItemNames"=w93) -> (error out=w90:errorcluster)  [unwired: 1 in, 1 out]
        n152 = case shown="True" w88 {
          tunnel: w90 -> [w107 w112]
          tunnel: [w107 w109] -> w86
          frame False {
          }
          frame True {
            n153 = property on="Wykres 1" class="WFGraph (strict)"(error in=w112) -> (error out=w111:errorcluster, "CrsrList"=w108:T13)  [unwired: 1 in, 1 out]
            n154 = property on="Wykres 2" class="WFGraph (strict)"(error in=w111, "CrsrList"=w108) -> (error out=w110:errorcluster)  [unwired: 1 in, 1 out]
            n155 = property on="Wykres 3" class="WFGraph (strict)"(error in=w110, "CrsrList"=w108) -> (error out=w109:errorcluster)  [unwired: 1 in, 1 out]
          }
        }
        n156 = call "Zapamietaj LogAdr.vi"() -> ("Log out"=w82:path)  [unwired: 8 in, 3 out]
        n157 = call "Log Error.vi"("base path"=w82, "Source"="Edycja", "error in"=w86) -> ("error out"=w85:errorcluster)  [unwired: 8 in]
        "Wykres 1" <- w79
        "Wykres 2" <- w79
        "Wykres 3" <- w79
      }
      n158 = local write "Tab Control"(T5."1 wykres" ("Tab Control")) -> ()
      n159 = control-ref of="Wykres 1"() -> (w54:refnum<vi>)
      n160 = property class="WFGraph (strict)"(reference=w54, error in=w62, "Value"=waveform(dbl)[] []) -> (error out=w61:errorcluster)  [unwired: 1 out]
    }
    frame Error {
    }
  }
  "error out" <- w7
  n161 = property on="error in (no error)" class="Clust (strict)"("Visible"=w4) -> ()  [unwired: 2 in, 2 out]
  n162 = property on="error out" class="Clust (strict)"("Visible"=w4) -> ()  [unwired: 2 in, 2 out]
  n163 = property on="Data in" class="Clust (strict)"("Visible"=w4) -> ()  [unwired: 2 in, 2 out]
  n164 = property on="Array" class="Arr (strict)"("Visible"=w4) -> ()  [unwired: 2 in, 2 out]
  n165 = property on="Zablokowane free out" class="Arr (strict)"("Visible"=w4) -> ()  [unwired: 2 in, 2 out]
  n166 = property on="Wykres 2" class="WFGraph (strict)"("Visible"=w3) -> ()  [unwired: 2 in, 2 out]
